vi "Find_LoginUser.vi"(3 "Login":T1, 4 "error in":errorcluster caption="에러 입력(에러 없음)", 7 "Root of UserList File":path=path "C:/Users/Administrator/Desktop/뻐꾸기/VI Library/SubVIs/Login/User.ini") -> (0 "error out":errorcluster caption="에러 출력")   [LabVIEW 2014]
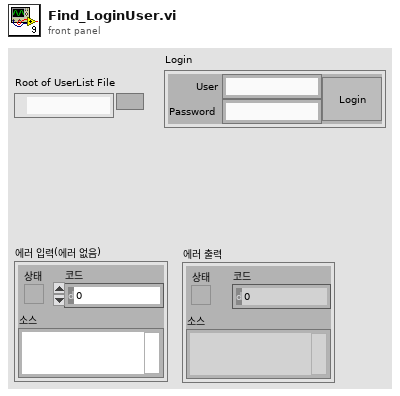
[diagram p1: front panel]
types:
  T1 = cluster{"User":string, "Password":string, "Login":bool}
  T2 = cluster{"section":string, "key":string, "value":string}[]
  T3 = cluster{"section":string, "key":string, "value":string}
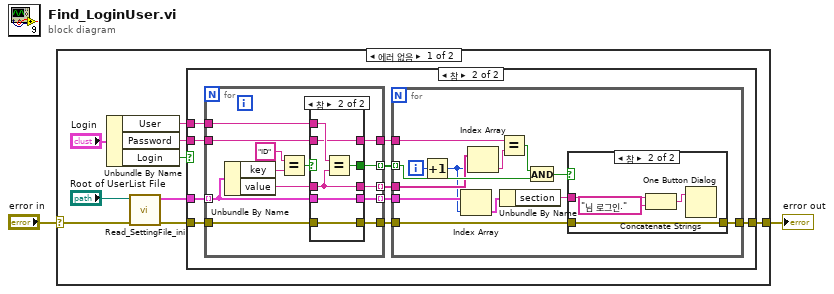
[diagram p0: block diagram]
diagram:
  n1 = case shown="에러 없음" "error in" {
    selector: "error in" -> [w11 w65]
    tunnel: [w3 w65] -> w1
    frame No Error {
      n2 = Unbundle By Name("Login") -> ("User"=w6:string, "Password"=w5:string, "Login"=w9:bool)
      n3 = call "Read_SettingFile_ini.vi"("error in"=w11, "Root of Setting File"="Root of UserList File") -> ("error out"=w7:errorcluster, "Settings"=w8:T2)  [unwired: 4 in]
      n4 = case shown="참" w9 {
        tunnel: w8 -> [_ w22]
        tunnel: w7 -> [w12 w19]
        tunnel: w6 -> [_ w21]
        tunnel: w5 -> [_ w20]
        tunnel: [w12 w13] -> w3
        frame False {
        }
        frame True {
          n5 = for {
            tunnel: w22 -> [w49] mode=indexing
            tunnel: w21 -> [w48]
            tunnel: w20 -> [w47]
            tunnel: [w42] -> w16
            tunnel: w19 -> [w51]
            tunnel: [w45] -> w14 mode=indexing
            tunnel: [w44] -> w17 mode=indexing
            tunnel: [w43] -> w15
            tunnel: [w41] -> w18 mode=indexing
            n6 = Unbundle By Name(w49) -> ("key"=w52:string, "value"=w46:string)
            n7 = Equal?(x="ID" ("key"), y=w52) -> (x = y?=w50:bool)
            n8 = case shown="참" w50 {
              selector: w50 -> [w55 _]
              tunnel: w51 -> [w56 w60]
              tunnel: w49 -> [w58 w63]
              tunnel: w48 -> [_ w64]
              tunnel: w47 -> [w57 w61]
              tunnel: w46 -> [w54 w59]
              tunnel: [w58 w63] -> w45
              tunnel: [w55 w62] -> w44
              tunnel: [w57 w61] -> w43
              tunnel: [w56 w60] -> w42
              tunnel: [w54 w59] -> w41
              frame False {
              }
              frame True {
                n9 = Equal?(x=w64, y=w59) -> (x = y?=w62:bool)
              }
            }
          }
          n10 = for {
            tunnel: w18 -> [w32]
            tunnel: w17 -> [w33] mode=indexing
            tunnel: w16 -> [w26]
            tunnel: w15 -> [w35]
            tunnel: w14 -> [w30]
            tunnel: [w23] -> w13
            i -> [w28]
            n11 = Increment(x=w28) -> (x+1=w27:i32)
            n12 = Index Array(array=w30, index=w27) -> (element=w29:T3)
            n13 = Index Array(array=w32, index=w27) -> (element=w31:string)
            n14 = Equal?(x=w35, y=w31) -> (x = y?=w34:bool)
            n15 = Unbundle By Name(w29) -> ("section"=w25:string)
            n16 = And(x=w34, y=w33) -> (x .and. y?=w24:bool)
            n17 = case shown="참" w24 {
              tunnel: w26 -> [w36 w37]
              tunnel: w25 -> [_ w39]
              tunnel: [w36 w37] -> w23
              frame False {
              }
              frame True {
                n18 = Concatenate Strings(w39, "님 로그인." ("문자열")) -> (w40:string)
                n19 = One Button Dialog(message=w40) -> ()  [unwired: 1 in, 1 out]
              }
            }
          }
        }
      }
    }
    frame Error {
    }
  }
  "error out" <- w1
